vi "Finish.vi"(8 "error in (no error)":errorcluster, 11 "Comp XBox One Controller in":refnum<class "Comp XBox One Controller.lvclass">) -> (0 "error out":errorcluster, 3 "Comp XBox One Controller out":refnum<class "Comp XBox One Controller.lvclass">)   [LabVIEW 2014, in "Comp XBox One Controller.lvlib" / "Comp XBox One Controller.lvclass"]
uses:
  Comp XBox One Controller.lvclass
  Comp XBox One Controller.lvclass/Comp XBox One Controller.ctl
  Robot/Xbox One Controller/XBox One Controller Class/XBox One Controller.lvclass
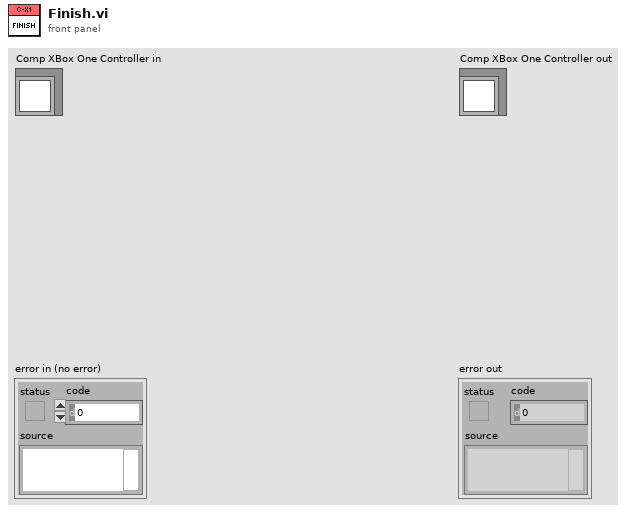
[diagram p1: front panel]
types:
  T1 = typedef "WPI_JoystickDevRef.ctl" = cluster{"Device":T2}
  T2 = typedef "WPI_JoystickDeviceEnum.ctl" = enum16{"USB 0", "USB 1", "USB 2", "USB 3", "USB 4", "USB 5"}
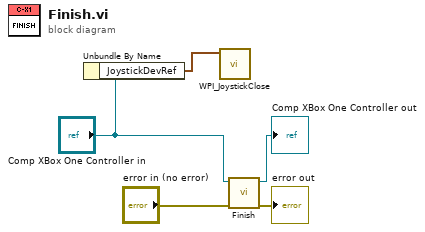
[diagram p0: block diagram]
diagram:
  n1 = Unbundle By Name("Comp XBox One Controller in") -> ("JoystickDevRef"=w1:T1)
  n2 = call <vilib>:"WPI_JoystickClose.vi"("JoystickDevRef"=w1) -> ()  [unwired: 11 in]
  n3 = call-parent "Finish.vi"("error in (no error)"="error in (no error)", "System Actor in"="Comp XBox One Controller in") -> ("error out"=→"error out":errorcluster, "System Actor out"=→"Comp XBox One Controller out":refnum<class "Comp XBox One Controller.lvclass">)  [unwired: 8 in]
